vi "Build Data Pointer.vi"(7 "Virtual Memory Unit in":refnum<class "Virtual Memory Unit.lvclass">, 8 "error in (no error)":errorcluster, 10 "Starting Address":u16 format="%04x", 11 "Message in":refnum<class "Message.lvclass">) -> (0 "error out":errorcluster, 2 "Next Available Address":u16 format="%04x", 3 "Message out":refnum<class "Message.lvclass">, 5 "Virtual Memory Unit out":refnum<class "Virtual Memory Unit.lvclass">)   [LabVIEW 2020, in "BCI-1553 API.lvlib" / "Message.lvclass"]
doc: "Writes the expected address for the message data into memory. This address will most certainly be following this block immediately."
uses:
  Message.lvclass
  Dependencies/Virtual Memory Unit/Virtual Memory Unit.lvclass
  BCI-1553 API.lvlib
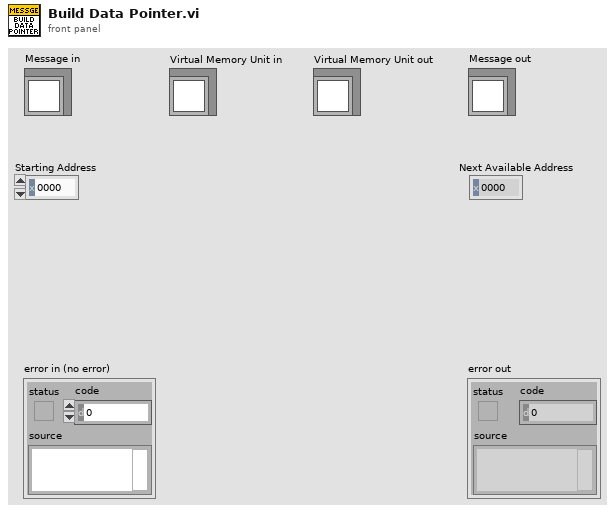
[diagram p1: front panel]
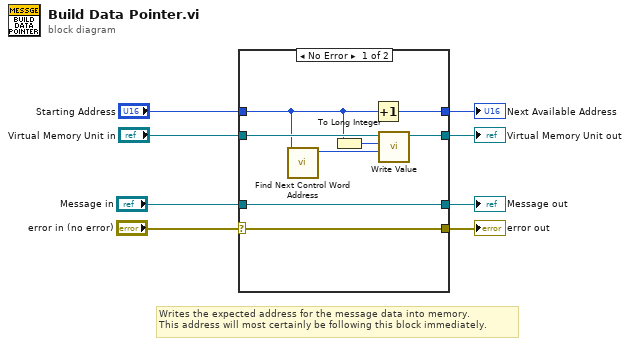
[diagram p0: block diagram]
diagram:
  # "Writes the expected address for the message data into memory.\nThis address will most certainly be following this block immediately."
  n1 = case shown="No Error" "error in (no error)" {
    selector: "error in (no error)" -> [w16 w20]
    tunnel: [w16 w20] -> w7
    tunnel: [w11 w19] -> w5
    tunnel: "Message in" -> [w11 w19]
    tunnel: "Starting Address" -> [w10 w18]
    tunnel: "Virtual Memory Unit in" -> [w14 w17]
    tunnel: [w15 w18] -> w2
    tunnel: [w13 w17] -> w1
    frame No Error {
      n2 = call "Find Next Control Word Address.vi"("Starting Address"=w10) -> ("0xHHHX Address"=w9:u16)  [unwired: 10 in]
      n3 = To Long Integer(number=w10) -> (32bit integer=w12:i32)
      n4 = Increment(x=w10) -> (x+1=w15:u16)
      n5 = call "Write Value.vi"("Value"=w9, "Index"=w12, "Virtual Memory Unit in"=w14) -> ("Virtual Memory Unit out"=w13:refnum<class "Virtual Memory Unit.lvclass">)  [unwired: 7 in, 1 out]
    }
    frame Error {
    }
  }
  "error out" <- w7
  "Message out" <- w5
  "Virtual Memory Unit out" <- w1
  "Next Available Address" <- w2
